vi "Exercises_7-1-2.vi"() -> ()   [LabVIEW 2014]
panel:
  out "error out":errorcluster
  in  "error in (no error)":errorcluster
  out "Warning?":bool
  out "Warning Text":string
  in  "Min Temp":dbl
  in  "Max Temp":dbl
  in  "Current Temp":dbl
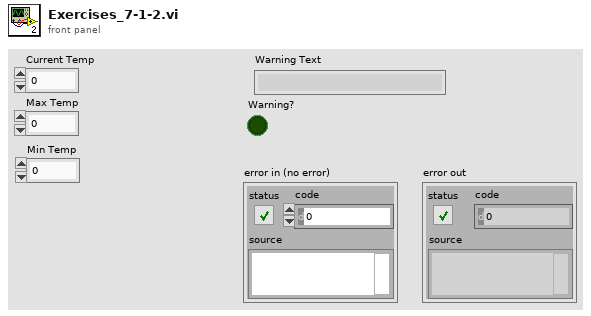
[diagram p1: front panel]
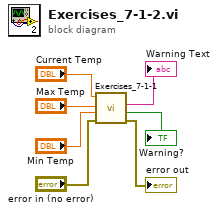
[diagram p0: block diagram]
diagram:
  n1 = call "Exercises_7-1-1.vi"("error in (no error)"="error in (no error)", "Min Temp"="Min Temp", "Max Temp"="Max Temp", "Current Temp"="Current Temp") -> ("error out"=→"error out":errorcluster, "Warning?"=→"Warning?":bool, "Warning Text"=→"Warning Text":string)  [unwired: 5 in]
